vi "getPIDgains.vi"() -> (0 "PID psi":T1={"proportional gain (Kc)"=0.5, "integral time (Ti, min)"=0.0, "derivative time (Td, min)"=0.0}, 1 "PID y":T1={"proportional gain (Kc)"=0.5, "integral time (Ti, min)"=0.0, "derivative time (Td, min)"=0.0}, 2 "PID x":T1={"proportional gain (Kc)"=0.5, "integral time (Ti, min)"=0.0, "derivative time (Td, min)"=0.0})   [LabVIEW 2014]
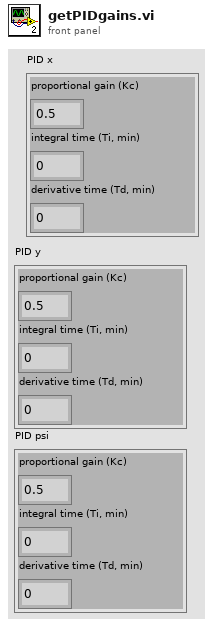
[diagram p1: front panel]
types:
  T1 = cluster{"proportional gain (Kc)":dbl, "integral time (Ti, min)":dbl, "derivative time (Td, min)":dbl}
  T2 = cluster{"Numeric":dbl, "Numeric 2":dbl, "Numeric 3":dbl}
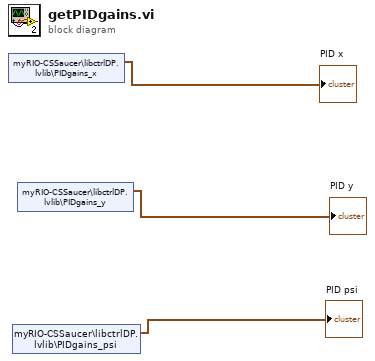
[diagram p0: block diagram]
diagram:
  n1 = shared-variable "myRIO-CSSaucer\\libctrlDP.lvlib\\PIDgains_x"() -> (→"PID x":T2)  [unwired: 1 in, 1 out]
  n2 = shared-variable "myRIO-CSSaucer\\libctrlDP.lvlib\\PIDgains_psi"() -> (→"PID psi":T2)  [unwired: 1 in, 1 out]
  n3 = shared-variable "myRIO-CSSaucer\\libctrlDP.lvlib\\PIDgains_y"() -> (→"PID y":T2)  [unwired: 1 in, 1 out]
